vi "DriveForTime-C.vi"(11 "Params":string[][](array[string])) -> ()   [LabVIEW 2017]
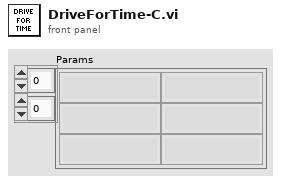
[diagram p1: front panel]
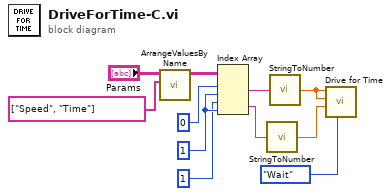
[diagram p0: block diagram]
diagram:
  w4 = 1
  n1 = call "ArrangeValuesByName.vi"("Names"=string[] ["Speed", "Time"], "Names/Values in"="Params") -> ("Names/Values Out"=w6:string[][])  [unwired: 9 in]
  n2 = Index Array(array=w6, index (row) #1=0, index (col) #1=w4, index (row) #2=1, index (col) #2=w4) -> (element #1=w2:string, element #2=w1:string)
  n3 = call "StringToNumber.vi"("String"=w1) -> ("Output"=w10:dbl)
  n4 = call "StringToNumber.vi"("String"=w2) -> ("Output"=w11:dbl)
  n5 = call "Drive for Time.vi"("Synchronization"=enum16{"Start", "Wait"}."Wait", "Seconds"=w10, "Right Speed"=w11, "Left Speed"=w11) -> ()  [unwired: 6 in, 2 out]
